vi "FindClassPath.vi"(8 "error in (no error)":errorcluster, 11 "Class Name":string) -> (0 "error out":errorcluster, 2 "Found?":bool, 3 "Class Path":path)   [LabVIEW 2019, in "Hawkeye.lvlib"]
uses:
  Hawkeye.lvlib
  <vilib>/SLL Toolkit/SLL String/SLL String.lvlib
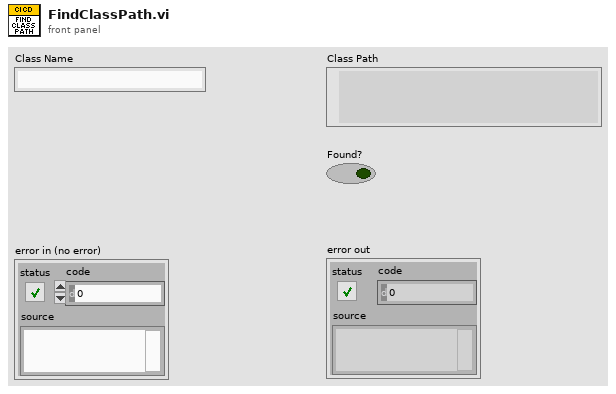
[diagram p1: front panel]
types:
  T1 = typedef "Hawkeye.lvlib/CICDPathConfigs.ctl" = cluster{"GlobalIncludePaths":path[], "GlobalExcludePaths":path[], "BuildSpecsIncludePaths":path[], "ActualDepsIncludePaths":path[], "WorkspacePath":path, "SourceFolderPaths":path[], "ChangedFilesLogpaths":map{string, path}}
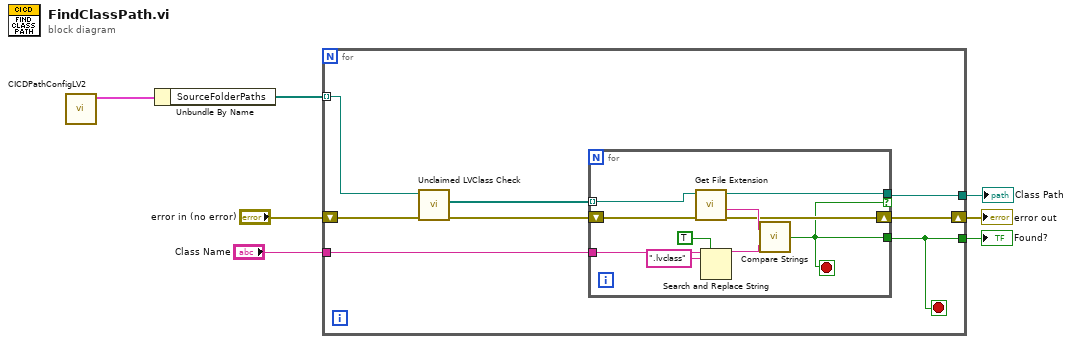
[diagram p0: block diagram]
diagram:
  n1 = call "CICDPathConfigLV2.vi"() -> ("CICD Path Config Out"=w2:T1)  [unwired: 11 in]
  n2 = Unbundle By Name(w2) -> ("SourceFolderPaths"=w1:path[])
  n3 = for {
    tunnel: [w15] -> w6
    tunnel: [w12] -> w5
    tunnel: "Class Name" -> [w14]
    shift-right: [w13] -> w3
    shift-left: "error in (no error)" -> [w9]
    tunnel: w1 -> [w10] mode=indexing
    stop <- w12 stop-if-true
    n4 = call "Unclaimed LVClass Check.vi"("error in (no error)"=w9, "Source Folder Path"=w10) -> ("error out"=w8:errorcluster, "Not owned (outside .lvlib)"=w11:path[])  [unwired: 6 in, 2 out]
    n5 = for {
      tunnel: w11 -> [w24] mode=indexing
      tunnel: w14 -> [w23]
      shift-right: [w18] -> w13
      shift-left: w8 -> [w25]
      tunnel: [w17] -> w15 if=w16
      tunnel: [w16] -> w12
      stop <- w16 stop-if-true
      n6 = call <vilib>:"Get File Extension.vi"("error in (no error)"=w25, "file"=w24) -> ("error out"=w18:errorcluster, "filename without extension"=w20:string, "dup file"=w17:path)  [unwired: 5 in, 2 out]
      n7 = Search and Replace String(replace all?=TRUE ("replace all? (F)"), input string=w23, search string=".lvclass") -> (result string=w19:string)  [unwired: 5 in, 3 out]
      n8 = call <vilib>:"Compare Strings.vi"("y"=w19, "x"=w20) -> ("Equal?"=w16:bool)
    }
  }
  "Class Path" <- w6
  "Found?" <- w5
  "error out" <- w3
